vi "AbstractNode_Create.vi"(0 "reference":refnum<class "AbstractNode.lvclass">, 5 "error in (no error)":errorcluster) -> (14 "reference out":refnum<class "AbstractNode.lvclass">, 19 "error out":errorcluster)   [LabVIEW 2014, in "AbstractNode.lvclass"]
doc: "Creates and initializes a new AbstractNode object.\n\nThis object should be destroyed using a AbstractNode destructor VI.\n\n[GOOP 2.1]"
uses:
  <resource>/Framework/Providers/Open_GDS/UML/AbstractNode_class/AbstractNode.lvclass
panel:
  # "The input reference should only\nbe wired when this method is called\nby a sub class constructor."
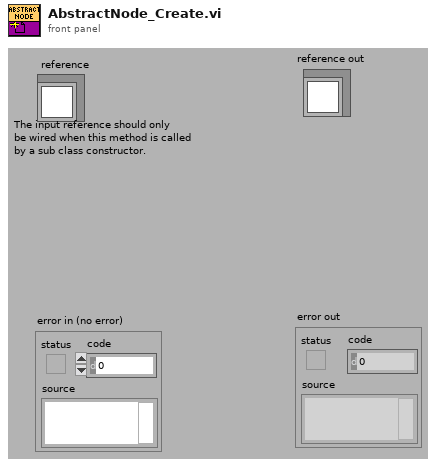
[diagram p1: front panel]
types:
  T1 = typedef "AbstractNode.lvclass/ObjectAttributes.ctl" = cluster{"parent":refnum<class "AbstractNode.lvclass">, "children":refnum<class "AbstractNode.lvclass">[], "Hidden":bool}
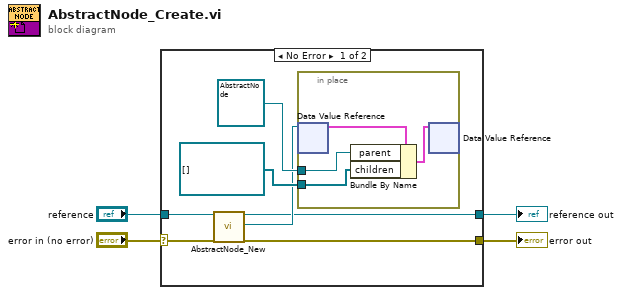
[diagram p0: block diagram]
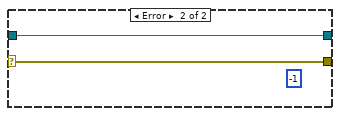
[diagram p2: hidden frame]
diagram:
  n1 = case shown="No Error" "error in (no error)" {
    selector: "error in (no error)" -> [w11 w17]
    tunnel: [w6 w16] -> w4
    tunnel: [w5 w17] -> w3
    tunnel: "reference" -> [w10 w16]
    frame No Error {
      n2 = call <resource>:"AbstractNode_New.vi"("reference in"=w10, "error in (no error)"=w11) -> ("reference out"=w6:refnum<class "AbstractNode.lvclass">, "DVRRefOut"=w7:refnum<data-value>, "error out"=w5:errorcluster)  [unwired: 2 in, 13 out]
      n3 = in-place {
        in-place-border: refnum<class "AbstractNode.lvclass"> refnum ("parent") -> [w14]
        in-place-border: refnum<class "AbstractNode.lvclass">[] [] ("children") -> [w13]
        n4 = in-place-dvr #1(w7) -> (w15:T1)  [unwired: 1 out]
        n5 = Bundle By Name(cluster=w15, "parent"=w14, "children"=w13) -> (w12:T1)
        n6 = in-place-dvr #1(w12) -> ()  [unwired: 2 out]
      }
    }
    frame Error {
      (unwired) -1 ("Nr of open handles")
    }
  }
  "error out" <- w3
  "reference out" <- w4
